vi "ConvertFloatToInt.vi"(1 "Variable Format":enum16{"INT", "FLOAT", "FIXED"}(ring), 2 "To Send in":string) -> (0 "To Send out":string)   [LabVIEW 2014]
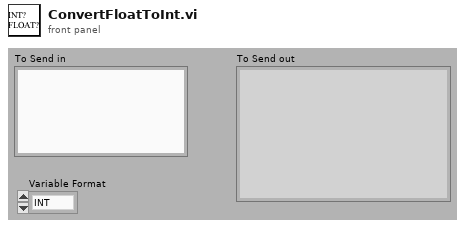
[diagram p1: front panel]
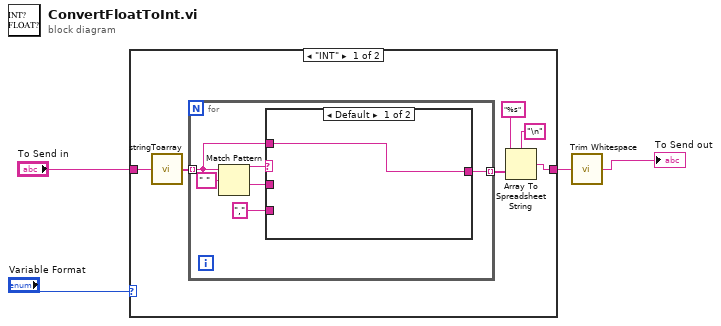
[diagram p0: block diagram]
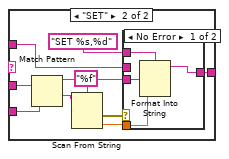
[diagram p2: hidden frame]
diagram:
  n1 = case shown="\"INT\"" "Variable Format" {
    tunnel: [w8 w33] -> w3
    tunnel: "To Send in" -> [w10 w33]
    frame "INT" {
      n2 = call <userlib>:"stringToarray.vi"("String"=w10) -> ("Array"=w9:string[])
      n3 = for {
        tunnel: w9 -> [w13] mode=indexing
        tunnel: [w11] -> w5 mode=indexing
        n4 = Match Pattern(string=w13, regular expression=" ") -> (before substring=w15:string, after substring=w12:string)  [unwired: 1 in, 2 out]
        n5 = case shown="Default" w15 {
          tunnel: "," ("regular expression") -> [_ w27]
          tunnel: [w17 w20] -> w11
          tunnel: w13 -> [w17 w19]
          tunnel: w12 -> [_ w18]
          frame Default {
          }
          frame "SET" {
            n6 = Match Pattern(string=w18, regular expression=w27) -> (before substring=w21:string, after substring=w26:string)  [unwired: 1 in, 2 out]
            n7 = Scan From String(format string="%f", input string=w26) -> (error out=w24:errorcluster, output 1=w22:dbl)  [unwired: 3 in, 2 out]
            n8 = case shown="No Error" w24 {
              tunnel: "SET %s,%d" ("regular expression") -> [w31 _]
              tunnel: w22 -> [w30 _]
              tunnel: w21 -> [w29 _]
              tunnel: [w28 w32] -> w20
              tunnel: w19 -> [_ w32]
              frame No Error {
                n9 = Format Into String(format string=w31, w29, w30) -> (resulting string=w28:string)  [unwired: 2 in, 1 out]
              }
              frame Error {
              }
            }
          }
        }
      }
      n10 = Array To Spreadsheet String(delimiter (Tab)="\n", array=w5, 3:"%s" ("format string")) -> (spreadsheet string=w8:string)
    }
    frame Default {
    }
  }
  n11 = call <vilib>:"Trim Whitespace.vi"("string"=w3) -> ("trimmed string"=→"To Send out":string)  [unwired: 1 in]
